vi "Joystick.vi"(2 "Multiplier":dbl=1.0, 3 "Input":dbl) -> (0 "In Dead Zone":bool, 1 "Output":dbl)   [LabVIEW 2013]
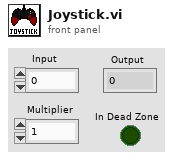
[diagram p1: front panel]
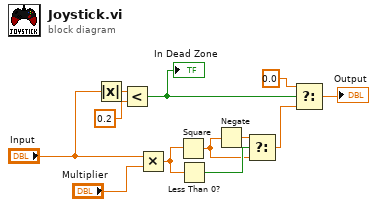
[diagram p0: block diagram]
diagram:
  n1 = Absolute Value(x="Input") -> (abs(x)=w6:dbl)
  n2 = Less?(x=w6, y=0.2) -> (x < y?=w3:bool)
  "In Dead Zone" <- w3
  n3 = Multiply(x="Input", y="Multiplier") -> (x*y=w7:dbl)
  n4 = Square(x=w7) -> (x^2=w10:dbl)
  n5 = Less Than 0?(x=w7) -> (x < 0?=w12:bool)
  n6 = Negate(x=w10) -> (-x=w11:dbl)
  n7 = Select(t=w11, s=w12, f=w10) -> (s? t:f=w2:dbl)
  n8 = Select(t=0.0, s=w3, f=w2) -> (s? t:f=→"Output":dbl)
